vi "Operator Loop.vi"() -> ()   [LabVIEW 2018]
uses:
  <vilib>/Platform/TimedLoop/XDataNode/wakeup.ctl
  <vilib>/Platform/TimedLoop/XDataNode/XDNodeRunTimeDep.lvlib
  <vilib>/Platform/TimedLoop/XDataNode/nitl_modes.ctl
  <vilib>/Platform/TimedLoop/XDataNode/timing_clust.ctl
  <vilib>/Platform/TimedLoop/XDataNode/XDataNode.xnode
  C:/Work/WRO/LidarCar/LidarCar/Operator Loop/Operator Loop Mode.ctl
panel:
  in  "outer threshold":dbl=1.1
  in  "inner threshold":dbl=0.6
  in  "max speed":dbl=0.4
  in  "stop?":bool
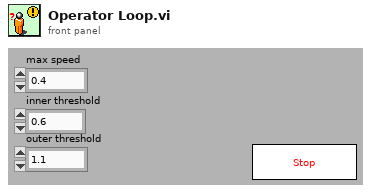
[diagram p1: front panel]
types:
  T1 = typedef "Operator Loop Mode.ctl" = enum16{"Idle", "Tele-Op", "Path Following", "Go Target", "Wall Correction", "Positioning", "Block Correction", "Get Color", "WhereGo", "Home Correction", "RC Control", "MoveTarget", "moveblock", "hands up", "hands down", "readQR"}
  T2 = typedef "XDNodeRunTimeDep.lvlib/timing_clust.ctl" = cluster{"Expected End [f-1]":u64, "Actual End [f-1]":u64, "Finished Late? [f-1]":bool, "Expected End [i-1]":u64, "Actual End [i-1]":u64, "Finished Late? [i-1]":bool, "Expected Start [i]":u64, "Actual Start [i]":u64, "Expected Start [f]":u64, "Actual Start [f]":u64, "Source Name":string, "Structure Name":string, "Period":i64, "Deadline":i64, "Offset":i64, "Start":i64, "Priority":i32, "Timeout":i32, "Mode":T3, "Wakeup Reason":T4, "Error":errorcluster, "Source Type":string, "Secondary Source Type":string, "Global End Time":u64, "Global Start Time":u64, "Frame Duration":u64, "Iteration Duration":u64, "Assigned CPU":i32, "I/O Scan Engine Mode":u32}
  T3 = typedef "XDNodeRunTimeDep.lvlib/nitl_modes.ctl" = enum32{"No Change", "Process missed periods, maintain original phase", "Discard missed periods, maintain original phase", "Process missed periods, ignore original phase", "Discard missed periods, ignore original phase"}
  T4 = typedef "XDNodeRunTimeDep.lvlib/wakeup.ctl" = enum32{"Normal", "Aborted", "Asynchronous wakeup", "Timing source error", "Timed loop error", "Timeout"}
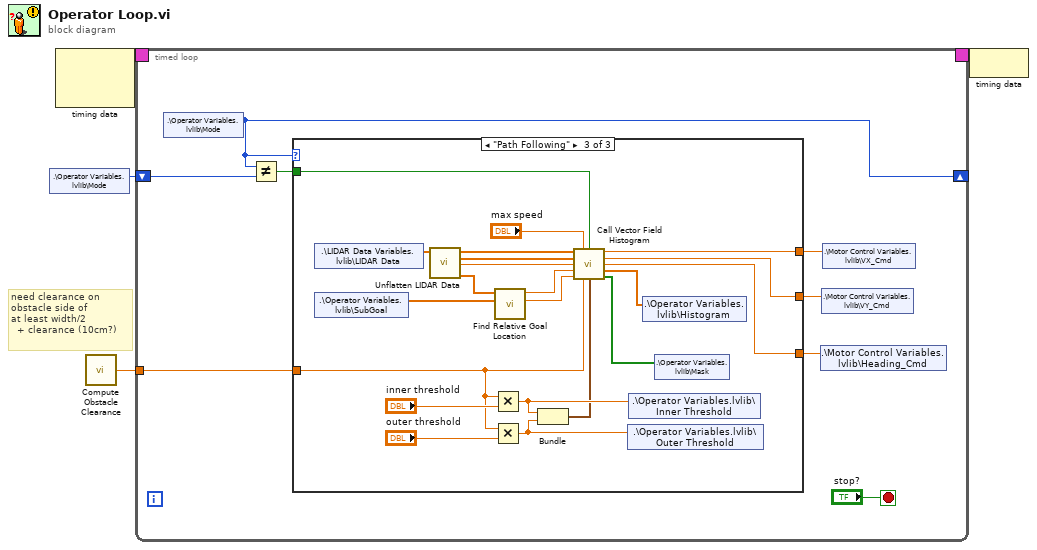
[diagram p0: block diagram]
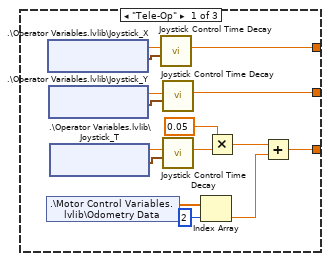
[diagram p2: hidden frame]
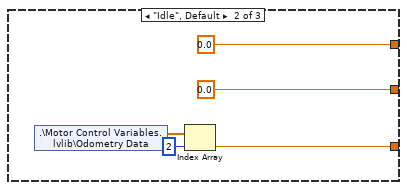
[diagram p3: hidden frame]
diagram:
  # "need clearance on \nobstacle side of \nat least width/2 \n  + clearance (10cm?)"
  n1 = shared-variable ".\\Operator Variables.lvlib\\Mode"() -> (w1:T1)  [unwired: 1 in, 1 out]
  n2 = node-c288() -> (w4:T2)  [unwired: 2 in]
  n3 = call "Compute Obstacle Clearance.vi"() -> ("obstacle clearance (m)"=w2:dbl)  [unwired: 1 in]
  n4 = timed-loop {
    timing: w4 -> [_]
    timing-out: [_] -> w3
    tunnel: w2 -> [w12]
    shift-right: [w5] -> _
    shift-left: w1 -> [w6]
    stop <- "stop?" stop-if-true
    n5 = shared-variable ".\\Operator Variables.lvlib\\Mode"() -> (w5:T1)  [unwired: 1 in, 1 out]
    n6 = Not Equal?(x=w5, y=w6) -> (x != y?=w7:bool)
    n7 = case shown="\"Path Following\"" w5 {
      tunnel: w12 -> [_ _ w42]
      tunnel: [w13 w28 w41] -> w10
      tunnel: [w19 0.0 ("Double") w34] -> w9
      tunnel: [w18 0.0 w35] -> w8
      tunnel: w7 -> [_ _ w49]
      frame "Tele-Op" {
        n8 = shared-variable ".\\Motor Control Variables.lvlib\\Odometry Data"() -> (w17:dbl[])  [unwired: 1 in, 1 out]
        n9 = shared-variable ".\\Operator Variables.lvlib\\Joystick_X"() -> (w21:dbl, w20:timestamp)  [unwired: 1 in, 1 out]
        n10 = shared-variable ".\\Operator Variables.lvlib\\Joystick_Y"() -> (w23:dbl, w22:timestamp)  [unwired: 1 in, 1 out]
        n11 = shared-variable ".\\Operator Variables.lvlib\\Joystick_T"() -> (w26:dbl, w25:timestamp)  [unwired: 1 in, 1 out]
        n12 = call "Joystick Control Time Decay.vi"("Time Stamp"=w20, "Value"=w21) -> ("Decayed Value"=w18:dbl)  [unwired: 9 in]
        n13 = call "Joystick Control Time Decay.vi"("Time Stamp"=w22, "Value"=w23) -> ("Decayed Value"=w19:dbl)  [unwired: 9 in]
        n14 = call "Joystick Control Time Decay.vi"("Time Stamp"=w25, "Value"=w26) -> ("Decayed Value"=w24:dbl)  [unwired: 9 in]
        n15 = Index Array(array=w17, index=2) -> (element=w15:dbl)
        n16 = Multiply(x=0.05 ("dtheta"), y=w24) -> (x*y=w14:dbl)
        n17 = Add(x=w14, y=w15) -> (x+y=w13:dbl)
      }
      frame "Idle", Default {
        n18 = shared-variable ".\\Motor Control Variables.lvlib\\Odometry Data"() -> (w30:dbl[])  [unwired: 1 in, 1 out]
        n19 = Index Array(array=w30, index=2) -> (element=w28:dbl)
      }
      frame "Path Following" {
        n20 = shared-variable ".\\LIDAR Data Variables.lvlib\\LIDAR Data"() -> (w52:dbl[])  [unwired: 1 in, 1 out]
        n21 = shared-variable ".\\Operator Variables.lvlib\\SubGoal"() -> (w53:dbl[])  [unwired: 1 in, 1 out]
        n22 = call "Unflatten LIDAR Data.vi"("Flat LIDAR Data"=w52) -> ("Robot Pose x,y (m)"=w48:dbl[], "Robot Pose Theta (rad)"=w40:dbl, "Bearing (rad)"=w50:dbl[], "Range (m)"=w51:dbl[])  [unwired: 7 in]
        n23 = Multiply(x=w42, y="inner threshold") -> (x*y=w38:dbl)
        n24 = Multiply(x=w42, y="outer threshold") -> (x*y=w37:dbl)
        n25 = call "Find Relative Goal Location.vi"("Goal Position"=w53, "Current Position"=w48) -> ("Target Distance"=w39:dbl, "Target Heading"=w33:dbl)  [unwired: 8 in]
        n26 = Bundle(w38, w37) -> (w36:cluster{dbl, dbl})  [unwired: 1 in]
        n27 = call "Call Vector Field Histogram.vi"("LIDAR magn. (m)"=w51, "max speed"="max speed", "Initialize?"=w49, "LIDAR angle (rad)"=w50, "current heading (rad)"=w40, "target heading (rad)"=w33, "target distance"=w39, "obstacle clearance (m)"=w42, "thresholds"=w36) -> ("command vx"=w35:dbl, "command vy"=w34:dbl, "command heading (rad)"=w41:dbl, "histogram out"=w44:dbl[], "mask out"=w43:bool[])  [unwired: 2 in]
        n28 = shared-variable ".\\Operator Variables.lvlib\\Outer Threshold"(w37) -> ()  [unwired: 1 in, 1 out]
        n29 = shared-variable ".\\Operator Variables.lvlib\\Inner Threshold"(w38) -> ()  [unwired: 1 in, 1 out]
        n30 = shared-variable ".\\Operator Variables.lvlib\\Histogram"(w44) -> ()  [unwired: 1 in, 1 out]
        n31 = shared-variable ".\\Operator Variables.lvlib\\Mask"(w43) -> ()  [unwired: 1 in, 1 out]
      }
    }
    n32 = shared-variable ".\\Motor Control Variables.lvlib\\Heading_Cmd"(w10) -> ()  [unwired: 1 in, 1 out]
    n33 = shared-variable ".\\Motor Control Variables.lvlib\\VY_Cmd"(w9) -> ()  [unwired: 1 in, 1 out]
    n34 = shared-variable ".\\Motor Control Variables.lvlib\\VX_Cmd"(w8) -> ()  [unwired: 1 in, 1 out]
  }
  n35 = node-c288(w3) -> ()
